vi "UpdateHistory.vi"(7 "CmbBox Refnum":refnum<vi>, 8 "Display State In 2":T1 caption="State", 11 "Data In":T2) -> (0 "Display State In":T1 caption="State")   [LabVIEW 2009, in "HistoryPath.xctl"]
uses:
  HistoryPath.xctl
  Data.ctl
  State.ctl
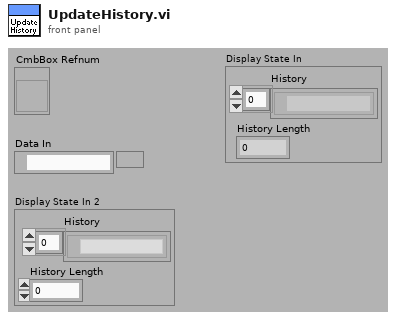
[diagram p1: front panel]
types:
  T1 = typedef "HistoryPath.xctl/State.ctl" = cluster{"History":path[], "History Length":i32}
  T2 = typedef "HistoryPath.xctl/Data.ctl" = path
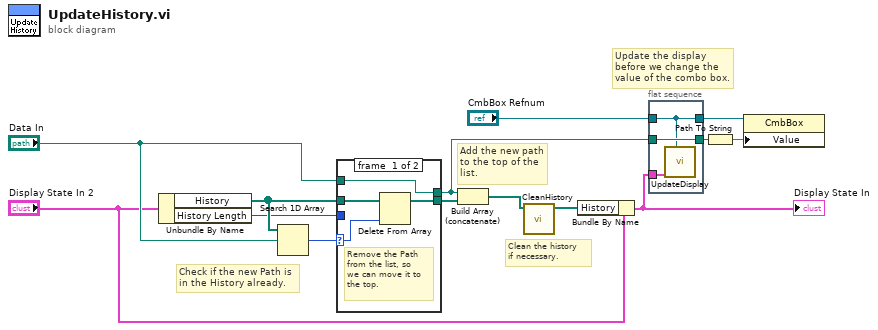
[diagram p0: block diagram]
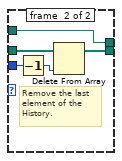
[diagram p2: hidden frame]
diagram:
  # "Update the display before we change the value of the combo box."
  # "Clean the history\nif necessary."
  # "Add the new path to the top of the\nlist."
  # "Check if the new Path is in the History already."
  n1 = Unbundle By Name("Display State In 2") -> ("History"=w11:path[], "History Length"=w9:i32)
  n2 = Search 1D Array(1D array=w11, element="Data In") -> (index of element=w13:i32)  [unwired: 1 in]
  n3 = case shown="0, Default" w13 {
    selector: w13 -> [w17 _]
    tunnel: w9 -> [_ w19]
    tunnel: [w16 w22] -> w14
    tunnel: w11 -> [w18 w23]
    tunnel: "Data In" -> [w15 w21]
    tunnel: [w15 w21] -> w5
    frame #0 {
      # "Remove the Path\nfrom the list, so\nwe can move it to\nthe top."
      n4 = Delete From Array(array=w18, index=w17) -> (array with subset deleted=w16:path[])  [unwired: 1 in, 1 out]
    }
    frame #1 {
      # "Remove the last\nelement of the\nHistory."
      n5 = Decrement(x=w19) -> (x-1=w20:i32)
      n6 = Delete From Array(array=w23, index=w20) -> (array with subset deleted=w22:path[])  [unwired: 1 in, 1 out]
    }
  }
  n7 = Build Array (concatenate)(w5, w14) -> (w2:T2[])
  n8 = call "CleanHistory.vi"("History Array In"=w2) -> ("History Array out"=w1:path[])  [unwired: 10 in]
  n9 = Bundle By Name(cluster="Display State In 2", "History"=w1) -> (w7:T1)
  "Display State In" <- w7
  n10 = flat-sequence {
    tunnel: w7 -> [w26]
    tunnel: "CmbBox Refnum" -> [w24]
    tunnel: [w25] -> w4
    tunnel: w5 -> [w25]
    tunnel: [w24] -> w3
    frame #0 {
      n11 = call "UpdateDisplay.vi"("CmbBox Refnum"=w24, "Display State In"=w26) -> ()  [unwired: 10 in]
    }
  }
  n12 = Path To String(path=w4) -> (string=w8:string)
  n13 = property on="Property Node" class="CmbBox"(reference=w3, "Value"=w8) -> ()  [unwired: 1 in, 2 out]
